vi "Lift Control.vi"(8 "bottom":bool, 9 "top":bool, 10 "Motor":dbl, 11 "Enum":T1) -> (3 "bottom switch on":bool)   [LabVIEW 2014]
uses:
  SRE Enum.ctl
  Text Variable VIs/Read Number Variable.vi
  <vilib>/Rock Robotics/WPI/MotorControl/WPI_MotorControlOpen Talon.vi
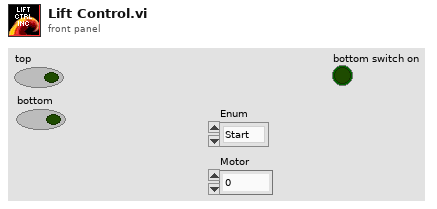
[diagram p1: front panel]
types:
  T1 = typedef "SRE Enum.ctl" = enum16{"Start", "Run", "End"}
  T2 = typedef "WPI_MotorControlDeviceRef.ctl" = cluster{"DeviceStatus":errorcluster, "Type":T3, "PWM":cluster{"Controller":T4, "PWM Channel":T5, "DeadBand":T6}, "CAN":cluster{"Device Number":u8, "Control Mode":T7, "Semaphore":T8, "Max Vout":dbl, "TalonSRX Control Mode":T9}, "Invert":bool, "TransformRef":T10, "InvTransformRef":T10}
  T3 = typedef "WPI_MotorControlType.ctl" = enum16{"PWM", "CAN", "CANTalonSRX"}
  T4 = typedef "FPGA_TypedefDigitalModule.ctl" = enum16{"Controller 1"}
  T5 = typedef "FPGA_DIOPWMChannel.ctl" = enum8{"PWM 0", "PWM 1", "PWM 2", "PWM 3", "PWM 4", "PWM 5", "PWM 6", "PWM 7", "PWM 8", "PWM 9", "PWM MXP 0", "PWM MXP 1", "PWM MXP 2", "PWM MXP 3", "PWM MXP 4", "PWM MXP 5", "PWM MXP 6", "PWM MXP 7", "PWM MXP 8", "PWM MXP 9", "Invalid"}
  T6 = typedef "WPI_PWMDeadband.ctl" = cluster{"Name":string, "maxPositivePwm":i32, "minPositivePwm":i32, "centerPwm":i32, "maxNegativePwm":i32, "minNegativePwm":i32, "angularRange":u16}
  T7 = typedef "WPI_CANJaguar_ControlMode.ctl" = enum8{"Percent VBus", "Current", "Speed", "Position", "Voltage"}
  T8 = typedef "Semaphore RefNum" = refnum<k1>
  T9 = typedef "WPI_CANTalonSRX_APIControlMode.ctl" = enum8{"Percent VBus", "Speed", "Position", "Slave", "Unchanged / Invalid"}
  T10 = typedef "WPI_PWMTransform_ConPane.ctl" = refnum<vi>
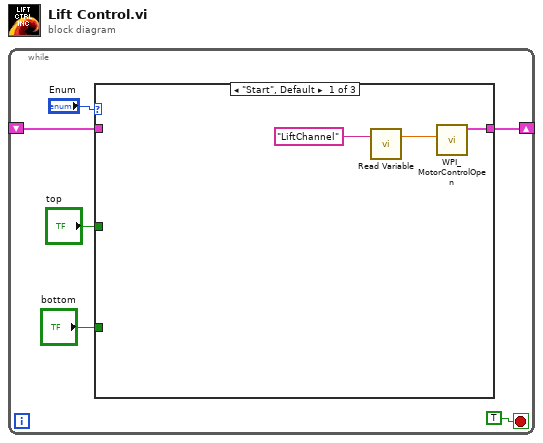
[diagram p0: block diagram]
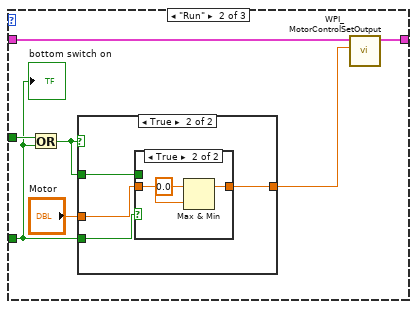
[diagram p2: hidden frame]
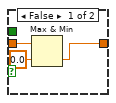
[diagram p4: hidden frame]
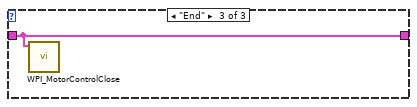
[diagram p5: hidden frame]
diagram:
  n1 = while {
    shift-right: [w5] -> _
    shift-left: _ -> [w4]
    stop <- TRUE stop-if-true
    n2 = case shown="\"Start\", Default" "Enum" {
      tunnel: [w7 w13 w28] -> w5
      tunnel: w4 -> [_ w12 w28]
      tunnel: "top" -> [_ w11 _]
      tunnel: "bottom" -> [_ w10 _]
      frame "Start", Default {
        n3 = call-poly "Read Variable.vi"("Name"="LiftChannel") -> ("number"=w8:dbl)  [unwired: 1 in, 1 out]
        n4 = call-poly <vilib>:"WPI_MotorControlOpen.vi"("PWM Channel"=w8) -> ("MotorControlDeviceRef"=w7:T2)  [unwired: 9 in, 1 out]
      }
      frame "Run" {
        n5 = Or(x=w11, y=w10) -> (x .or. y?=w16:bool)
        n6 = case shown="True" w16 {
          tunnel: w16 -> [_ w21]
          tunnel: "Motor" -> [w17 w20]
          tunnel: [w17 w19] -> w14
          tunnel: w10 -> [_ w18]
          frame False {
          }
          frame True {
            n7 = case shown="True" w18 {
              tunnel: w21 -> [_ _]
              tunnel: w20 -> [w24 w27]
              tunnel: [w22 w25] -> w19
              frame False {
                n8 = Max & Min(x=w24, y=0.0) -> (min(x,y)=w22:dbl)  [unwired: 1 out]
              }
              frame True {
                n9 = Max & Min(x=0.0, y=w27) -> (max(x,y)=w25:dbl)  [unwired: 1 out]
              }
            }
          }
        }
        n10 = call <vilib>:"WPI_MotorControlSetOutput.vi"("Output"=w14, "MotorControlDevRef"=w12) -> ("MotorControlDevRef"=w13:T2)  [unwired: 7 in, 2 out]
        "bottom switch on" <- w10
      }
      frame "End" {
        n11 = call <vilib>:"WPI_MotorControlClose.vi"("MotorControlDevRef"=w28) -> ()  [unwired: 10 in, 1 out]
      }
    }
  }
